vi "Init from Ref.vi"(8 "error in":errorcluster, 10 "CellContext .NET":refnum<k24>) -> (0 "error out":errorcluster, 3 "Cell Context out":refnum<class "Cell Context.lvclass">)   [LabVIEW 2024, in "SourceGrid.lvlib" / "Cell Context.lvclass"]
uses:
  Cell Context.lvclass
  D:/git/Sourcegrid-LabVIEW/dll/SourceGrid.dll
  dll/SourceGrid.dll
  Cell Context.lvclass/Cell Context.ctl
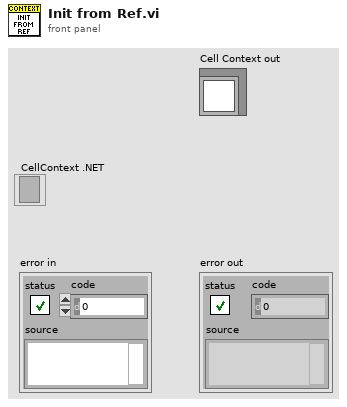
[diagram p1: front panel]
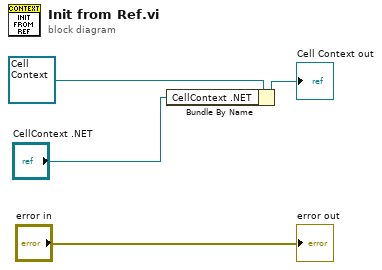
[diagram p0: block diagram]
diagram:
  n1 = Bundle By Name(cluster=refnum<class "Cell Context.lvclass"> refnum ("Cell Context in"), "CellContext .NET"="CellContext .NET") -> (→"Cell Context out":refnum<class "Cell Context.lvclass">)
  "error out" <- "error in"
